vi "CtrlTreeAddParentNode.vi"(8 "error in (no error)":errorcluster, 9 "Prefix":string, 10 "Parent Tag":string, 11 "TreeControl in":refnum<vi>) -> (0 "error out":errorcluster, 2 "Tag out":string, 3 "TreeControl out":refnum<vi>)   [LabVIEW 2021]
uses:
  CtrlTreeAddItemIndent.vi
  CtrlTreeAddItemParent.vi
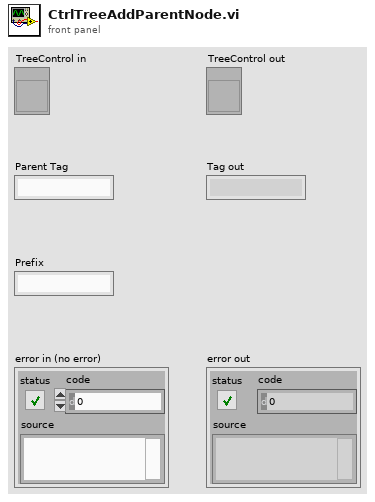
[diagram p1: front panel]
types:
  T1 = cluster{"string array[0]":string, "string array[1]":string, "string array[2]":string}
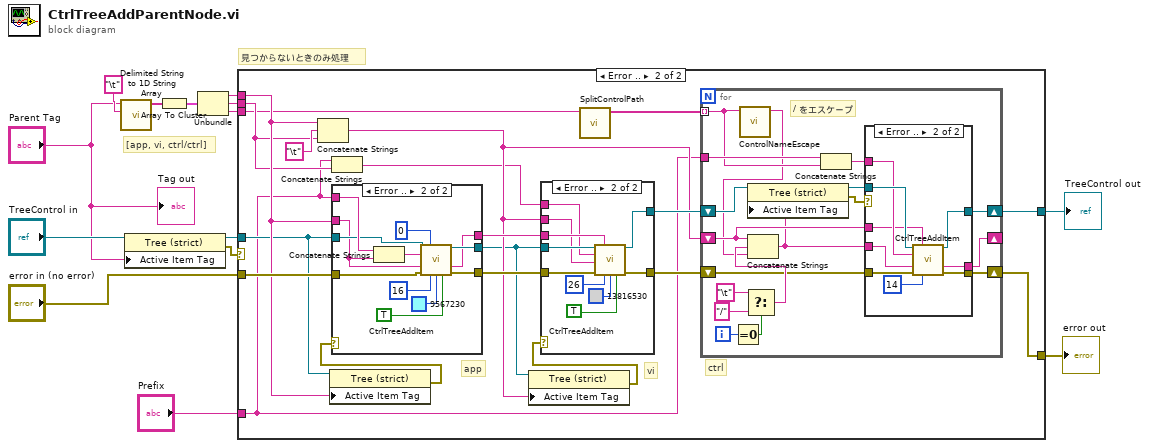
[diagram p0: block diagram]
diagram:
  # "[app, vi, ctrl/ctrl]"
  # "見つからないときのみ処理"
  n1 = call <vilib>:"Delimited String to 1D String Array.vi"("delimiter"="\t", "delimited string"="Parent Tag") -> ("string array"=w7:string[])  [unwired: 9 in]
  n2 = property class="Tree (strict)"(reference="TreeControl in", "Active Item Tag"="Parent Tag") -> (reference out=w11:refnum<vi>, error out=w9:errorcluster)  [unwired: 1 in]
  n3 = Array To Cluster(array=w7) -> (cluster=w8:T1)
  n4 = Unbundle(w8) -> ("string array[0]"=w5:string, "string array[1]"=w4:string, "string array[2]"=w3:string)
  n5 = case shown="Error .." w9 {
    tunnel: [w16 w29] -> w13
    tunnel: [w15 w24] -> w12
    tunnel: w11 -> [w16 w22]
    tunnel: "error in (no error)" -> [w15 w33]
    tunnel: w5 -> [_ w26]
    tunnel: w4 -> [_ w25]
    tunnel: w3 -> [_ w18]
    tunnel: "Prefix" -> [_ w19]
    frame No Error {
    }
    frame Error {
      # "app"
      # "ctrl"
      # "vi"
      n6 = Concatenate Strings(w26, "\t" ("delimiter"), w25) -> (w23:string)
      n7 = property class="Tree (strict)"(reference=w22, "Active Item Tag"=w26) -> (error out=w35:errorcluster)  [unwired: 1 in, 1 out]
      n8 = Concatenate Strings(w19, w25) -> (w21:string)
      n9 = case shown="Error .." w35 {
        tunnel: [w37 w43] -> w20
        tunnel: w22 -> [w37 w47]
        tunnel: w26 -> [w38 w42]
        tunnel: w19 -> [_ w50]
        tunnel: [w38 w41] -> w34
        tunnel: [w36 w40] -> w32
        tunnel: w33 -> [w36 w39]
        frame No Error {
        }
        frame Error {
          n10 = Concatenate Strings(w50, w42) -> (w48:string)
          n11 = call-poly "CtrlTreeAddItem.vi"("TreeControl in"=w47, "Indentation"=0, "Left Cell String"=w48, "Tag"=w42, "error in (no error)"=w39, "Symbol Index"=16, "Background Color"=u32 9567230, "Bold Font"=TRUE) -> ("TreeControl out"=w43:refnum<vi>, "Tag out"=w41:string, "error out"=w40:errorcluster)  [unwired: 5 in]
        }
      }
      n12 = property class="Tree (strict)"(reference=w20, "Active Item Tag"=w23) -> (error out=w31:errorcluster)  [unwired: 1 in, 1 out]
      n13 = case shown="Error .." w31 {
        tunnel: w34 -> [_ w55]
        tunnel: w21 -> [_ w54]
        tunnel: [w52 w59] -> w30
        tunnel: [w51 w58] -> w28
        tunnel: w20 -> [w52 w57]
        tunnel: w32 -> [w51 w56]
        tunnel: w23 -> [_ w53]
        frame No Error {
        }
        frame Error {
          n14 = call-poly "CtrlTreeAddItem.vi"("TreeControl in"=w57, "Parent Tag"=w55, "Left Cell String"=w54, "Tag"=w53, "error in (no error)"=w56, "Symbol Index"=26, "Background Color"=u32 13816530, "Bold Font"=TRUE) -> ("TreeControl out"=w59:refnum<vi>, "error out"=w58:errorcluster)  [unwired: 5 in, 1 out]
        }
      }
      n15 = call "SplitControlPath.vi"("control path string"=w18) -> ("string array"=w17:string[])  [unwired: 9 in, 1 out]
      n16 = for {
        tunnel: w17 -> [w64] mode=indexing
        shift-right: [w66] -> _
        shift-left: w23 -> [w71]
        shift-right: [w69] -> w29
        shift-left: w30 -> [w80]
        shift-right: [w67] -> w24
        shift-left: w28 -> [w68]
        tunnel: w19 -> [w65]
        i -> [w76]
        # "/ をエスケープ"
        n17 = Equal To 0?(x=w76) -> (x = 0?=w75:bool)
        n18 = call "ControlNameEscape.vi"("label"=w64) -> ("escaped string"=w63:string)  [unwired: 10 in]
        n19 = Select(t="\t", s=w75, f="/") -> (s? t:f=w72:string)
        n20 = Concatenate Strings(w71, w72, w63) -> (w70:string)
        n21 = property class="Tree (strict)"(reference=w80, "Active Item Tag"=w70) -> (reference out=w78:refnum<vi>, error out=w79:errorcluster)  [unwired: 1 in]
        n22 = Concatenate Strings(w65, w64) -> (w77:string)
        n23 = case shown="Error .." w79 {
          tunnel: w78 -> [w83 w92]
          tunnel: w77 -> [_ w91]
          tunnel: w70 -> [w81 w90]
          tunnel: w71 -> [_ w89]
          tunnel: [w83 w87] -> w69
          tunnel: w68 -> [w82 w86]
          tunnel: [w82 w85] -> w67
          tunnel: [w81 w84] -> w66
          frame No Error {
          }
          frame Error {
            n24 = call-poly "CtrlTreeAddItem.vi"("TreeControl in"=w92, "Parent Tag"=w89, "Left Cell String"=w91, "Tag"=w90, "error in (no error)"=w86, "Symbol Index"=14) -> ("TreeControl out"=w87:refnum<vi>, "Tag out"=w84:string, "error out"=w85:errorcluster)  [unwired: 7 in]
          }
        }
      }
    }
  }
  "TreeControl out" <- w13
  "error out" <- w12
  "Tag out" <- "Parent Tag"
